vi "Initial Connection.vi"(0 "Systems Config Path":path=path "C:/Users/gtetil/Documents/Projects/TI-cDAQ/Source/Systems Config.ini", 5 "Error IN":errorcluster) -> (14 "Close Program":bool, 15 "Connected":bool, 16 "System Ref":tag, 17 "Selected System":T1, 19 "Error OUT":errorcluster)   [LabVIEW 2023]
uses:
  Type Defs and Controls/System Buttons.ctl
  Type Defs and Controls/System Button.ctl
  Type Defs and Controls/System Config.ctl
  Type Defs and Controls/Systems Config.ctl
  <vilib>/Utility/cursorutil.llb/Set Cursor (Icon Pict).vi
  <vilib>/Utility/config.llb/NI_LVConfig.lvlib
  <userlib>/_OpenG.lib/variantconfig/variantconfig.llb/openg_variant_configuration_file.lvlib
panel:
  out "Abort 2":bool
  in  "Exit":bool
  in  "Abort":bool
  out "Connecting Indicator":string="Connecting..."
  in  "Tab Control":enum32{"Main", "Connecting"}(tab)
  in  "Systems":T2={"System 1"={"System Button"=FALSE, "Description"="Deformation"}, "System 2"={"System Button"=FALSE, "Description"="Standard"}, "System 3"={"System Button"=FALSE, "Description"="Standard"}, "System 4"={"System Button"=FALSE, "Description"="Standard"}, "System 5"={"System Button"=FALSE, "Description"="Standard XT"}, "System 6"={"System Button"=FALSE, "Description"=""}, "System 7"={"System Button"=FALSE, "Description"=""}, "System 8"={"System Button"=FALSE, "Description"=""}, "System 9"={"System Button"=FALSE, "Description"=""}}
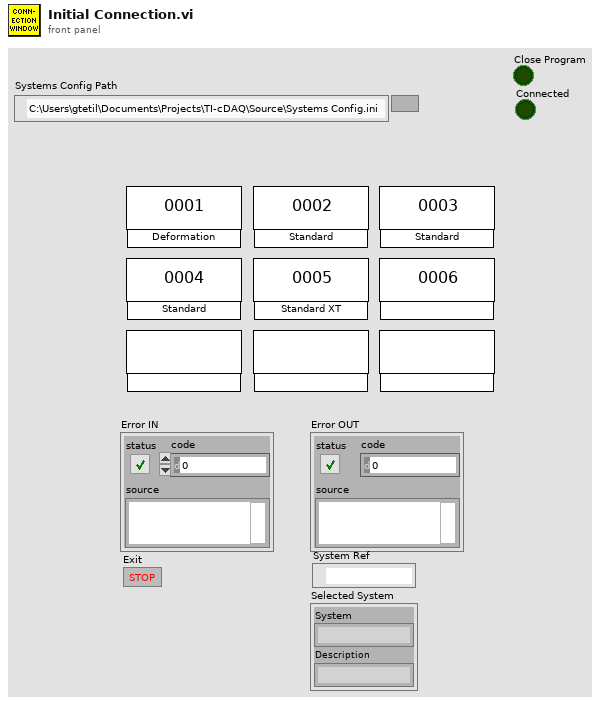
[diagram p1: front panel]
types:
  T1 = typedef "System Config.ctl" = cluster{"System":string, "Description":string}
  T2 = typedef "System Buttons.ctl" = cluster{"System 1":T3, "System 2":T3, "System 3":T3, "System 4":T3, "System 5":T3, "System 6":T3, "System 7":T3, "System 8":T3, "System 9":T3}
  T3 = typedef "System Button.ctl" = cluster{"System Button":bool, "Description":string}
  T4 = typedef "Systems Config.ctl" = cluster{"System 1":T1, "System 2":T1, "System 3":T1, "System 4":T1, "System 5":T1, "System 6":T1, "System 7":T1, "System 8":T1, "System 9":T1}
  T5 = cluster{"Error IN":errorcluster, "Systems Config Path":path, "Systems Config":T4, "Selected System":T1, "Close Program":bool, "Connected":bool, "System Ref":tag}
  T6 = enum8{"Enabled", "Disabled", "Disabled and Grayed Out"}
  T7 = typedef "NI_LVConfig.lvlib/Config Data RefNum.ctl" = refnum<k1>
  T8 = enum32{"invalid app kind", "Development System", "Run Time System", "Student Edition", "Embedded LabVIEW", "Evaluation", "Custom"}
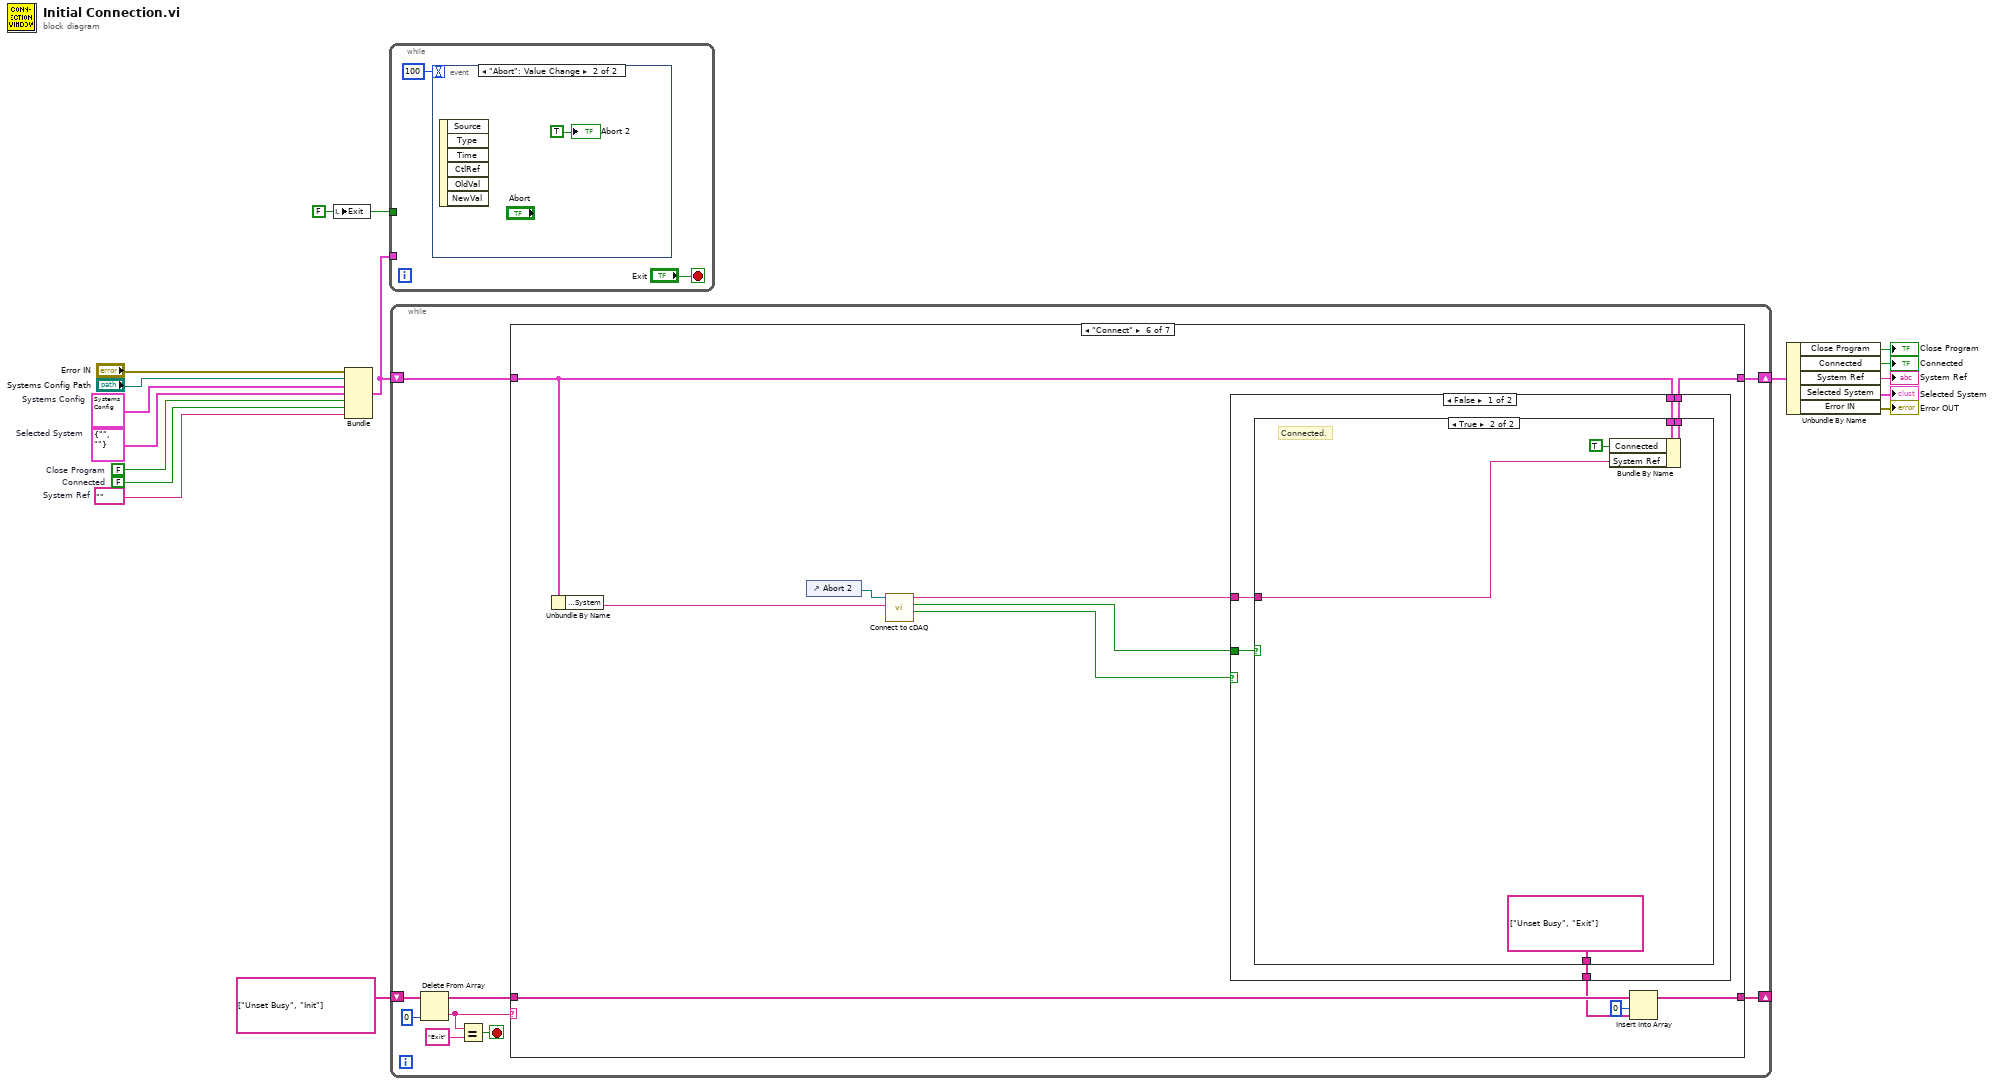
[diagram p0: block diagram]
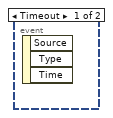
[diagram p2: hidden frame]
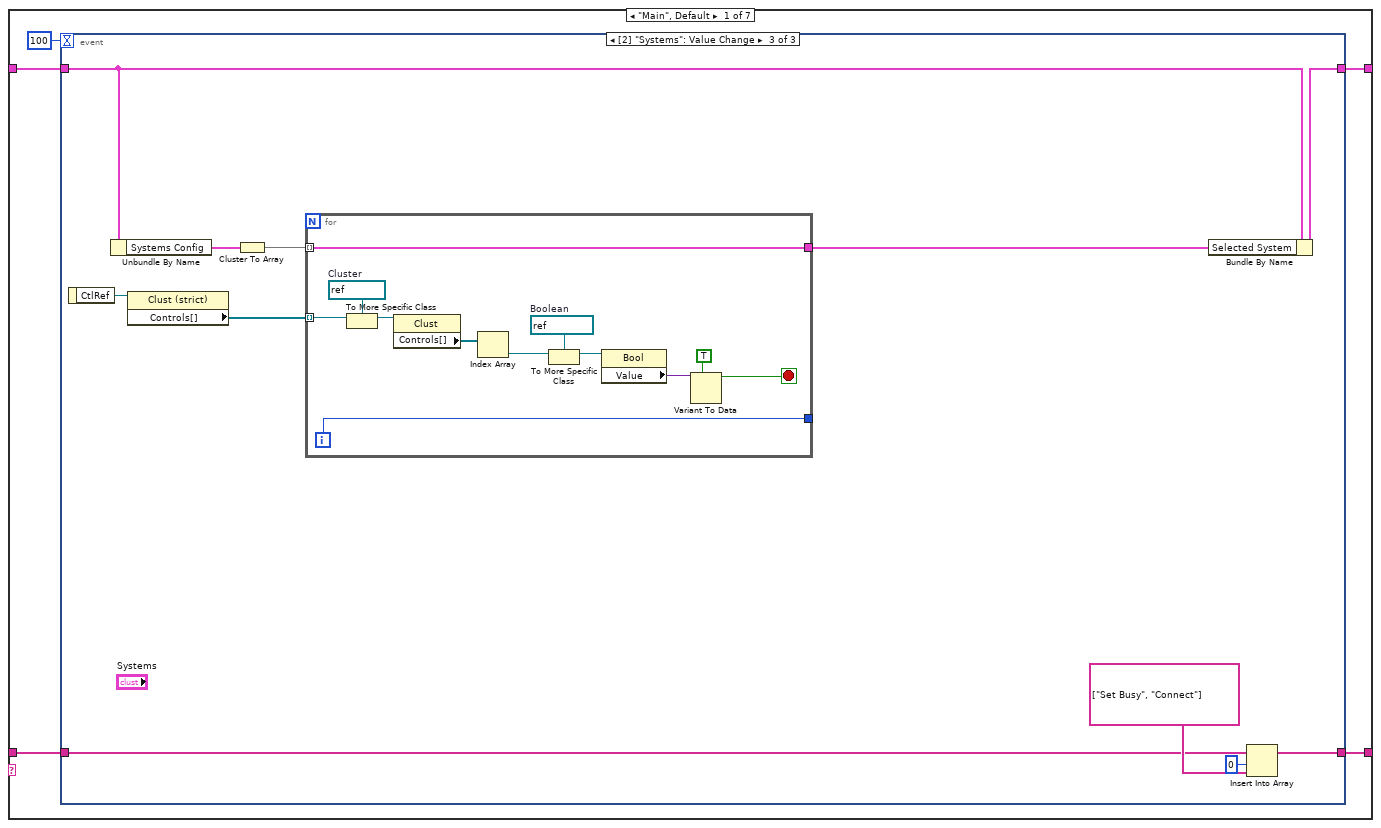
[diagram p3: hidden frame]
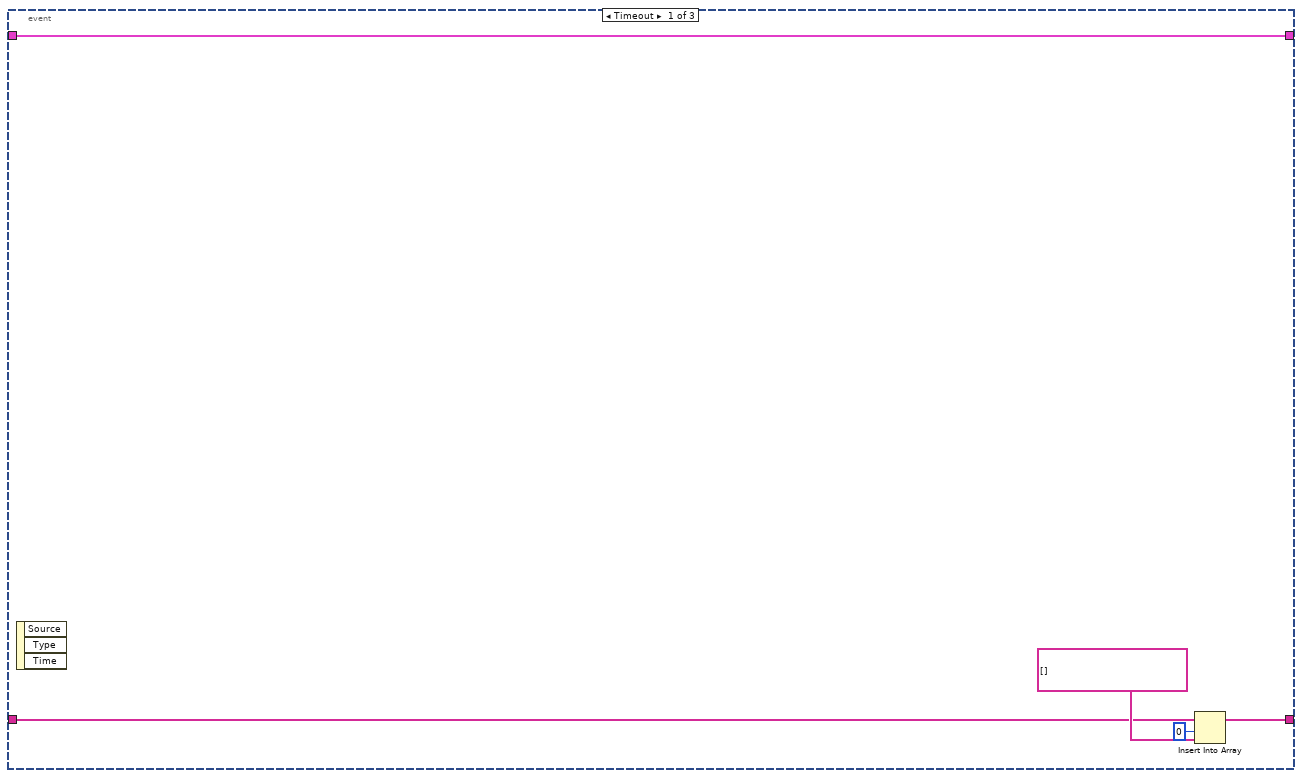
[diagram p4: hidden frame]
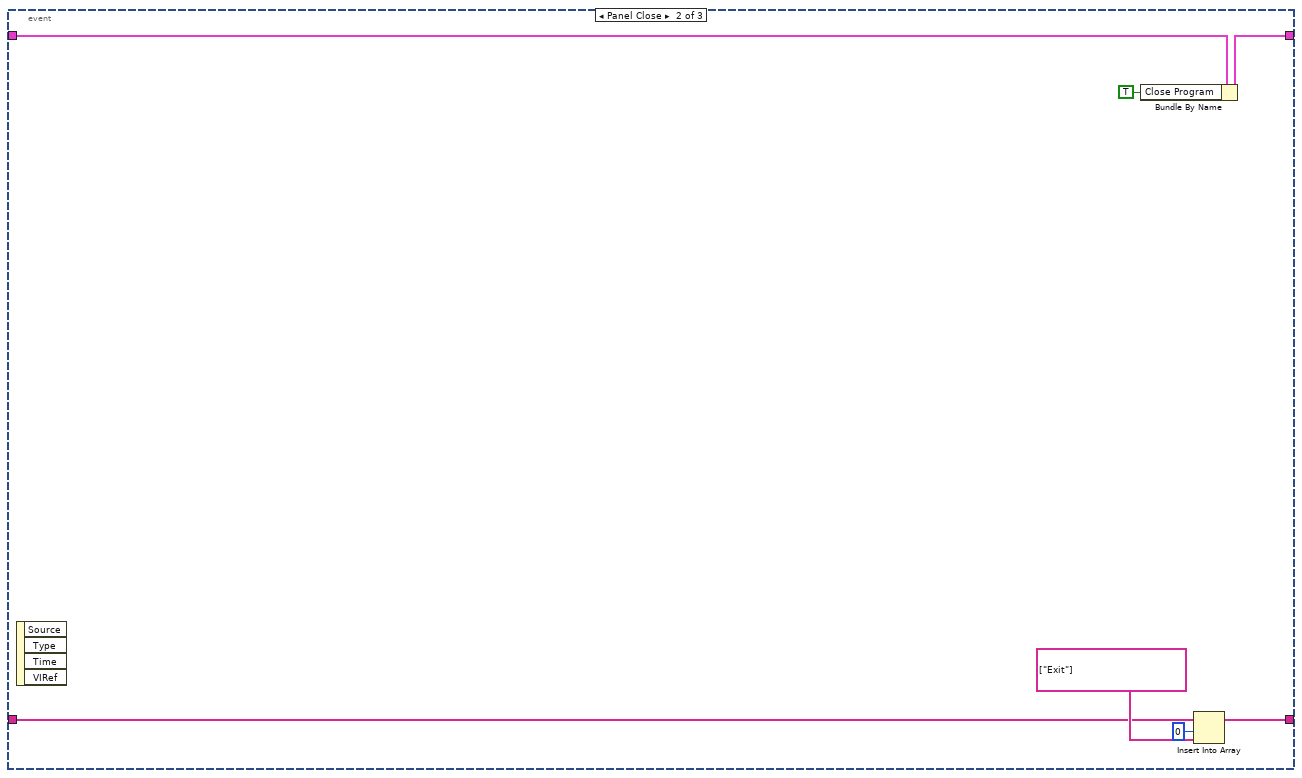
[diagram p5: hidden frame]
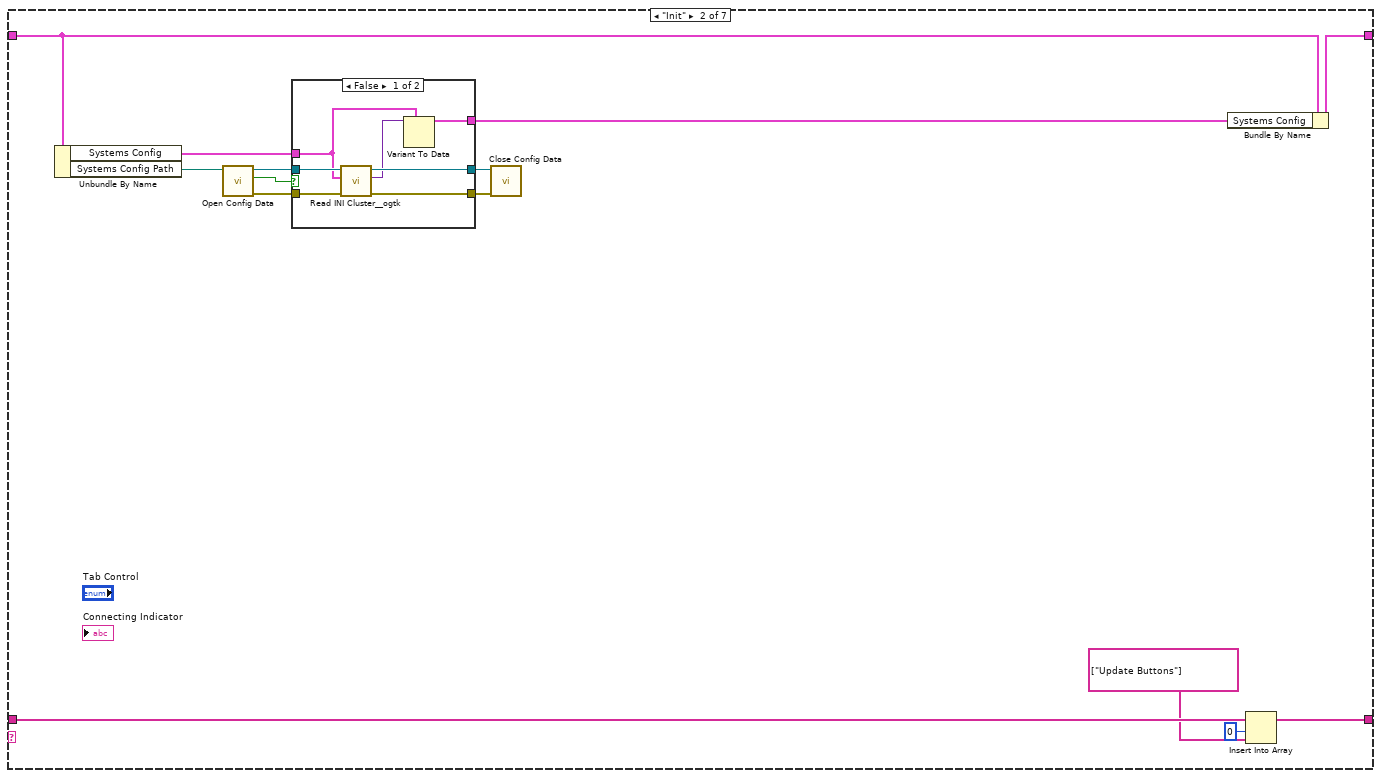
[diagram p6: hidden frame]
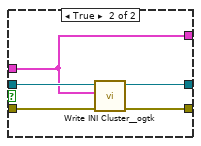
[diagram p7: hidden frame]
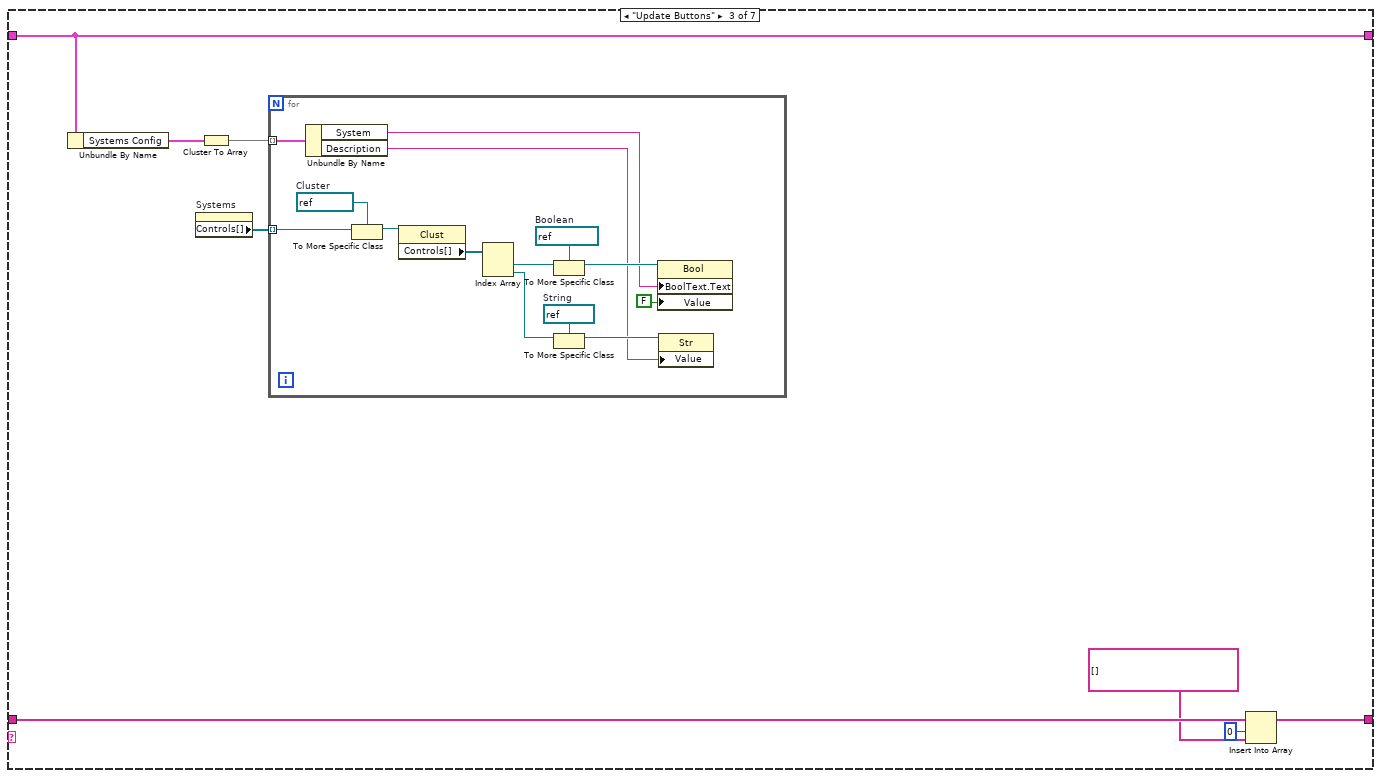
[diagram p8: hidden frame]
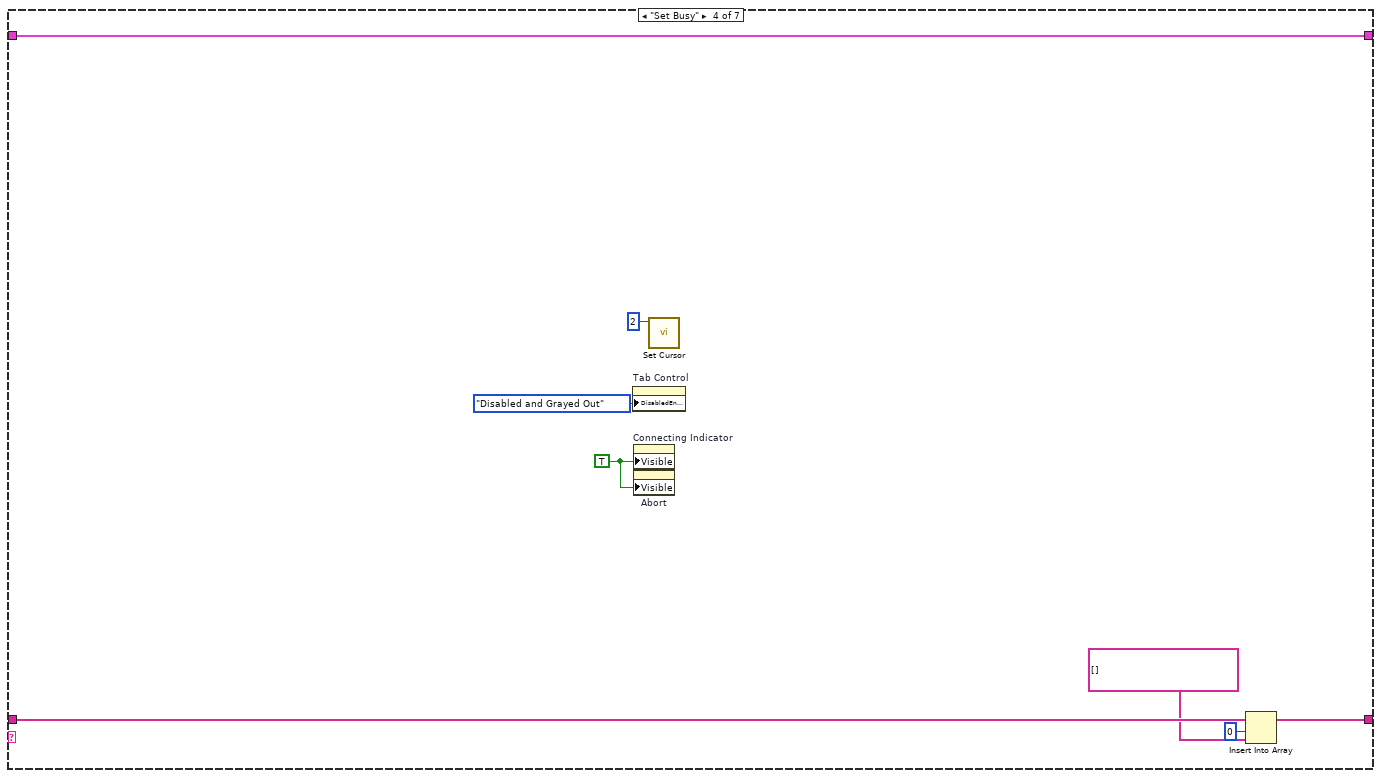
[diagram p9: hidden frame]
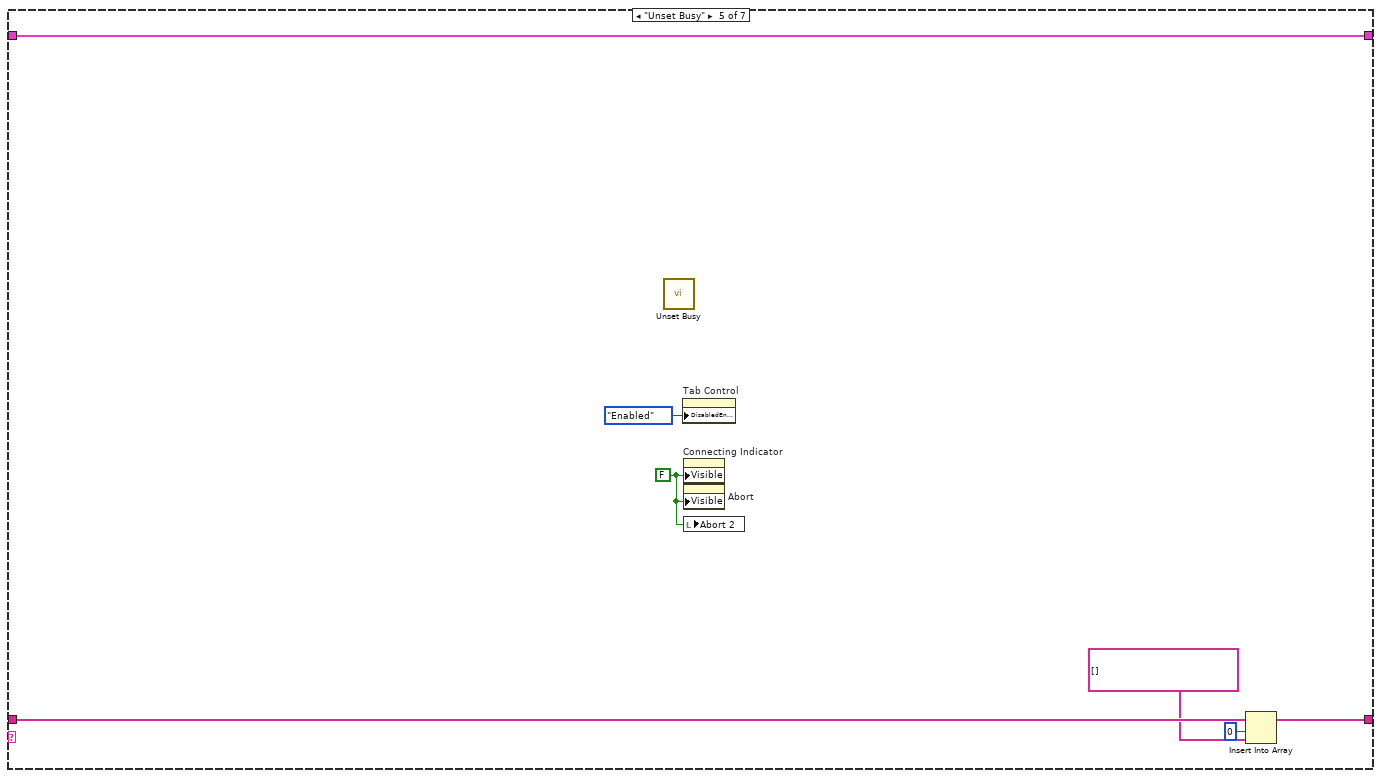
[diagram p10: hidden frame]
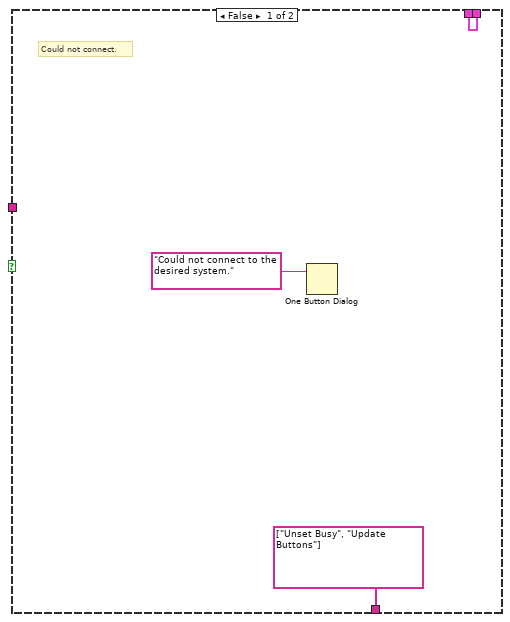
[diagram p11: hidden frame]
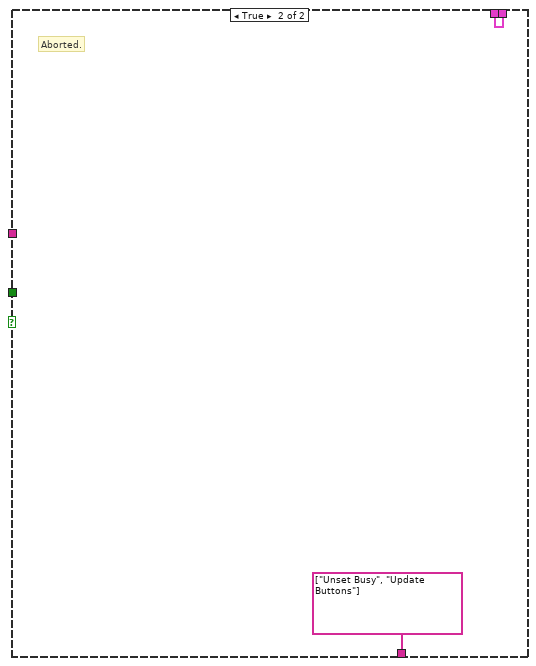
[diagram p12: hidden frame]
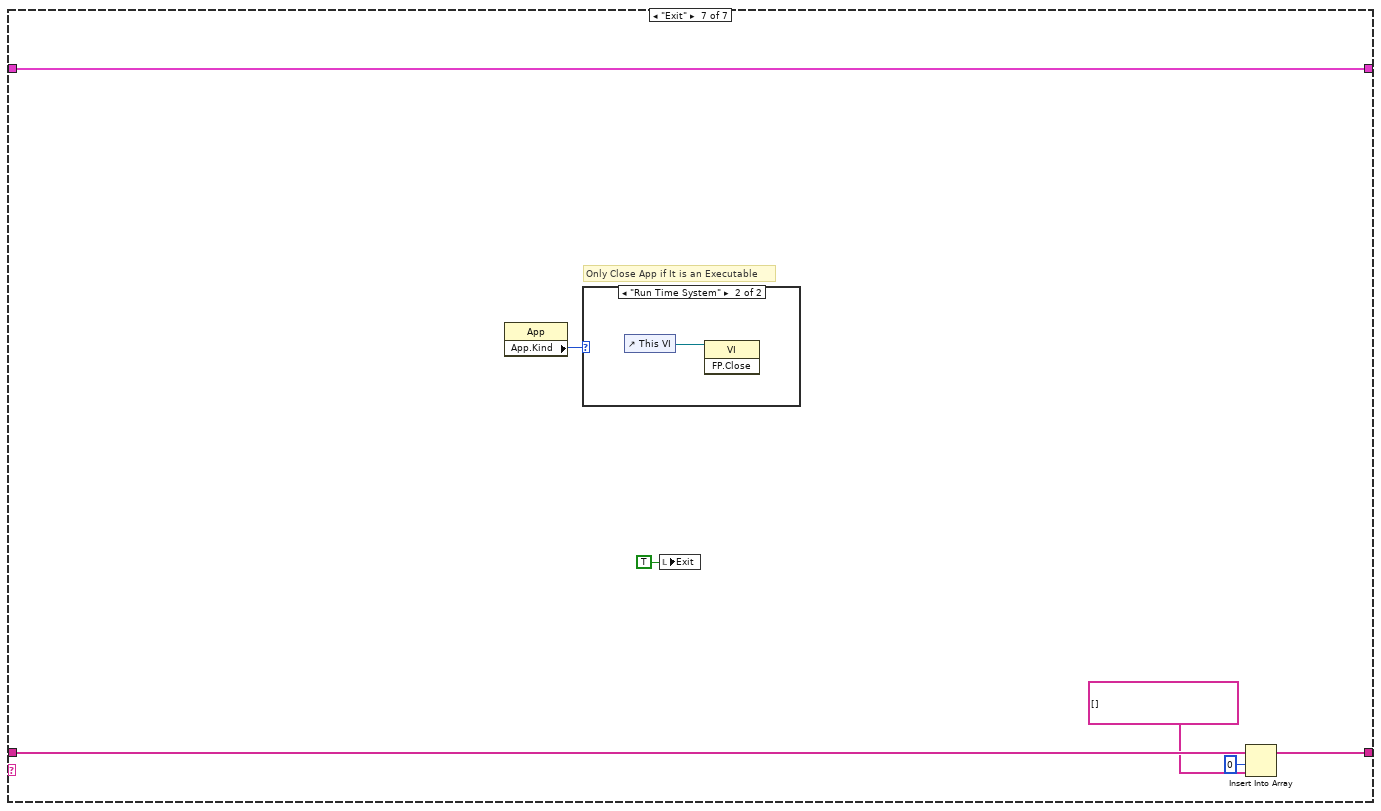
[diagram p13: hidden frame]
diagram:
  w1 = FALSE ("Exit")
  w5 = tag ""  # System Ref
  w8 = FALSE  # Connected
  w11 = FALSE  # Close Program
  w12 = T1 {"System"="", "Description"=""}  # Selected System
  w13 = T4 {"System 1"={"System"="", "Description"=""}, "System 2"={"System"="", "Description"=""}, "System 3"={"System"="", "Description"=""}, "System 4"={"System"="", "Description"=""}, "System 5"={"System"="", "Description"=""}, "System 6"={"System"="", "Description"=""}, "System 7"={"System"="", "Description"=""}, "System 8"={"System"="", "Description"=""}, "System 9"={"System"="", "Description"=""}}  # Systems Config
  n1 = local write "Exit"(w1) -> ()
  n2 = Bundle("Error IN"="Error IN", "Systems Config Path"="Systems Config Path", "Systems Config"=w13, "Selected System"=w12, "Close Program"=w11, "Connected"=w8, "System Ref"=w5) -> (w2:T5)  [unwired: 1 in]
  n3 = while {
    tunnel: w2 -> [_]
    tunnel: w1 -> [_]
    stop <- "Exit" stop-if-true
    n4 = event shown="[1] \"Abort\": Value Change" {
      selector: _ -> [_ _]
      dyn-events: _ -> [_ _]
      timeout: 100 -> [_ _]
      event Timeout {
        n5 = event-data() -> ()  [unwired: 1 in, 3 out]
      }
      event "Abort": Value Change {
        n6 = event-data() -> ()  [unwired: 1 in, 6 out]
        "Abort 2" <- TRUE ("Abort 2")
      }
    }
  }
  n7 = while {
    shift-right: [w23] -> _
    shift-left: string[] ["Unset Busy", "Init"] -> [w28]
    shift-right: [w20] -> w10
    shift-left: w2 -> [w21]
    stop <- w24 stop-if-true
    n8 = Delete From Array(array=w28, index=0 ("length")) -> (deleted portion=w25:string, array with subset deleted=w22:string[])  [unwired: 1 in]
    n9 = Equal?(x=w25, y="Exit") -> (x = y?=w24:bool)
    n10 = case shown="\"Connect\"" w25 {
      tunnel: [w29 w81 w102 w124 w131 w142 w164] -> w23
      tunnel: w22 -> [w30 w80 w101 w123 w130 w141 w163]
      tunnel: w21 -> [w33 w77 w98 w120 w127 w136 w160]
      tunnel: [w32 w82 w98 w120 w127 w137 w160] -> w20
      frame "Main", Default {
        n11 = event shown="[2] \"Systems\": Value Change" {
          selector: _ -> [_ _ _]
          dyn-events: _ -> [_ _ _]
          timeout: 100 -> [_ _ _]
          tunnel: w33 -> [w38 w40 w49]
          tunnel: [w38 w41 w50] -> w32
          tunnel: w30 -> [w35 w42 w54]
          tunnel: [w34 w43 w53] -> w29
          event Timeout {
            n12 = event-data() -> ()  [unwired: 1 in, 3 out]
            n13 = Insert Into Array(array=w35, index=0, new element=string[] []) -> (w34:string[])
          }
          event Panel Close {
            n14 = event-data() -> ()  [unwired: 1 in, 4 out]
            n15 = Bundle By Name(cluster=w40, "Close Program"=TRUE) -> (w41:T5)
            n16 = Insert Into Array(array=w42, index=0, new element=string[] ["Exit"]) -> (w43:string[])
          }
          event Value Change {
            n17 = event-data() -> ("CtlRef"=w52:refnum<vi>)  [unwired: 1 in]
            n18 = Unbundle By Name(w49) -> ("Systems Config"=w48:T4)
            n19 = property class="Clust (strict)"(reference=w52) -> ("Controls[]"=w51:refnum<vi>[])  [unwired: 1 in, 2 out]
            n20 = Cluster To Array(cluster=w48) -> (array=w47:T1[])
            n21 = for {
              tunnel: w51 -> [w62] mode=indexing
              tunnel: [w58] -> _
              tunnel: w47 -> [w57] mode=indexing
              tunnel: [w57] -> w46
              i -> [w58]
              stop <- w59 stop-if-true
              w64 = refnum<vi> refnum  # Boolean
              w63 = refnum<vi> refnum  # Cluster
              n22 = To More Specific Class(target class=w63, reference=w62) -> (specific class reference=w68:refnum<vi>)  [unwired: 1 in, 1 out]
              n23 = property class="Clust"(reference=w68) -> ("Controls[]"=w67:refnum<vi>[])  [unwired: 1 in, 2 out]
              n24 = Index Array(array=w67) -> (element=w66:refnum<vi>)  [unwired: 1 in]
              n25 = To More Specific Class(target class=w64, reference=w66) -> (specific class reference=w65:refnum<vi>)  [unwired: 1 in, 1 out]
              n26 = property class="Bool"(reference=w65) -> ("Value"=w61:variant)  [unwired: 1 in, 2 out]
              n27 = Variant To Data(type=TRUE, Variant=w61) -> (data=w59:bool)  [unwired: 1 in, 1 out]
            }
            n28 = Bundle By Name(cluster=w49, "Selected System"=w46) -> (w50:T5)
            n29 = Insert Into Array(array=w54, index=0, new element=string[] ["Set Busy", "Connect"]) -> (w53:string[])
          }
        }
      }
      frame "Init" {
        n30 = Unbundle By Name(w77) -> ("Systems Config"=w71:T4, "Systems Config Path"=w76:path)
        n31 = call <vilib>:"Open Config Data.vi"("configuration file path"=w76) -> ("error out"=w75:errorcluster, "file created?"=w69:bool, "refnum"=w74:T7)  [unwired: 8 in]
        n32 = case shown="False" w69 {
          tunnel: w75 -> [w89 w93]
          tunnel: w74 -> [w88 w94]
          tunnel: [w87 w92] -> w73
          tunnel: [w86 w91] -> w72
          tunnel: w71 -> [w85 w90]
          tunnel: [w83 w90] -> w70
          frame False {
            n33 = call <userlib>:"Read INI Cluster__ogtk.vi"("error in (no error)"=w89, "INI Fomatted Cluster Type"=w85, "refnum"=w88) -> ("error out"=w86:errorcluster, "INI Fomatted Cluster"=w84:variant, "dup refnum"=w87:T7)  [unwired: 4 in, 2 out]
            n34 = Variant To Data(type=w85, Variant=w84) -> (data=w83:T4)  [unwired: 1 in, 1 out]
          }
          frame True {
            n35 = call <userlib>:"Write INI Cluster__ogtk.vi"("error in (no error)"=w93, "INI Fomatted Cluster"=w90, "refnum"=w94) -> ("error out"=w91:errorcluster, "dup refnum"=w92:T7)  [unwired: 7 in]
          }
        }
        n36 = call <vilib>:"Close Config Data.vi"("error in (no error)"=w72, "refnum"=w73) -> ()  [unwired: 8 in, 2 out]
        n37 = Bundle By Name(cluster=w77, "Systems Config"=w70) -> (w82:T5)
        n38 = Insert Into Array(array=w80, index=0, new element=string[] ["Update Buttons"]) -> (w81:string[])
      }
      frame "Update Buttons" {
        n39 = Unbundle By Name(w98) -> ("Systems Config"=w97:T4)
        n40 = property on="Systems" class="Clust (strict)"() -> ("Controls[]"=w95:refnum<vi>[])  [unwired: 2 in, 2 out]
        n41 = Cluster To Array(cluster=w97) -> (array=w96:T1[])
        n42 = for {
          tunnel: w96 -> [w116] mode=indexing
          tunnel: w95 -> [w113] mode=indexing
          w109 = refnum<vi> refnum  # String
          w110 = refnum<vi> refnum  # Boolean
          w112 = refnum<vi> refnum  # Cluster
          n43 = Unbundle By Name(w116) -> ("System"=w105:string, "Description"=w104:string)
          n44 = To More Specific Class(target class=w112, reference=w113) -> (specific class reference=w115:refnum<vi>)  [unwired: 1 in, 1 out]
          n45 = property class="Clust"(reference=w115) -> ("Controls[]"=w114:refnum<vi>[])  [unwired: 1 in, 2 out]
          n46 = Index Array(array=w114) -> (element #1=w111:refnum<vi>, element #2=w108:refnum<vi>)  [unwired: 2 in]
          n47 = To More Specific Class(target class=w110, reference=w111) -> (specific class reference=w107:refnum<vi>)  [unwired: 1 in, 1 out]
          n48 = To More Specific Class(target class=w109, reference=w108) -> (specific class reference=w106:refnum<vi>)  [unwired: 1 in, 1 out]
          n49 = property class="Bool"(reference=w107, "BoolText.Text"=w105, "Value"=FALSE) -> ()  [unwired: 1 in, 2 out]
          n50 = property class="Str"(reference=w106, "Value"=w104) -> ()  [unwired: 1 in, 2 out]
        }
        n51 = Insert Into Array(array=w101, index=0, new element=string[] []) -> (w102:string[])
      }
      frame "Set Busy" {
        w118 = TRUE ("Visible")
        n52 = property on="Tab Control" class="TabCtl (strict)"("DisabledEnum"=T6."Disabled and Grayed Out" ("Disabled")) -> ()  [unwired: 2 in, 2 out]
        n53 = property on="Connecting Indicator" class="Str"("Visible"=w118) -> ()  [unwired: 2 in, 2 out]
        n54 = property on="Abort" class="Bool"("Visible"=w118) -> ()  [unwired: 2 in, 2 out]
        n55 = call-poly <vilib>:"Set Cursor.vi"("icon"=u16 2) -> ()  [unwired: 9 in, 2 out]
        n56 = Insert Into Array(array=w123, index=0, new element=string[] []) -> (w124:string[])
      }
      frame "Unset Busy" {
        w125 = FALSE ("Visible")
        n57 = call <vilib>:"Unset Busy.vi"() -> ()  [unwired: 11 in, 1 out]
        n58 = property on="Tab Control" class="TabCtl (strict)"("DisabledEnum"=T6."Enabled" ("Disabled")) -> ()  [unwired: 2 in, 2 out]
        n59 = property on="Connecting Indicator" class="Str"("Visible"=w125) -> ()  [unwired: 2 in, 2 out]
        n60 = property on="Abort" class="Bool"("Visible"=w125) -> ()  [unwired: 2 in, 2 out]
        n61 = local write "Abort 2"(w125) -> ()
        n62 = Insert Into Array(array=w130, index=0, new element=string[] []) -> (w131:string[])
      }
      frame "Connect" {
        n63 = Unbundle By Name(w136) -> ("Selected System.System"=w133:string)
        n64 = control-ref of="Abort 2"() -> (w132:refnum<vi>)
        n65 = call "Connect to cDAQ.vi"("System"=w133, "Abort Ref"=w132) -> ("Abort"=w134:bool, "Connected?"=w138:bool, "System Ref"=w135:tag)  [unwired: 7 in]
        n66 = case shown="False" w134 {
          tunnel: [w147 string[] ["Unset Busy", "Update Buttons"]] -> w140
          tunnel: w138 -> [w146 _]
          tunnel: [w145 w157] -> w137
          tunnel: w136 -> [w144 w157]
          tunnel: w135 -> [w143 _]
          frame False {
            n67 = case shown="True" w146 {
              tunnel: [string[] ["Unset Busy", "Update Buttons"] string[] ["Unset Busy", "Exit"]] -> w147
              tunnel: w144 -> [w150 w154]
              tunnel: [w150 w153] -> w145
              tunnel: w143 -> [_ w151]
              frame False {
                # "Could not connect."
                n68 = One Button Dialog(message="Could not connect to the desired system.") -> ()  [unwired: 1 in, 1 out]
              }
              frame True {
                # "Connected."
                n69 = Bundle By Name(cluster=w154, "Connected"=TRUE, "System Ref"=w151) -> (w153:T5)
              }
            }
          }
          frame True {
            # "Aborted."
          }
        }
        n70 = Insert Into Array(array=w141, index=0, new element=w140) -> (w142:string[])
      }
      frame "Exit" {
        # "Only Close App if It is an Executable"
        n71 = property class="App"() -> ("App.Kind"=w158:T8)  [unwired: 2 in, 2 out]
        n72 = case shown="\"Run Time System\"" w158 {
          frame Default {
          }
          frame "Run Time System" {
            n73 = control-ref of="This VI"() -> (w165:refnum<vi>)
            n74 = invoke class="VI" method="FP.Close"(reference=w165) -> ()  [unwired: 2 in, 3 out]
          }
        }
        n75 = local write "Exit"(TRUE ("Exit")) -> ()
        n76 = Insert Into Array(array=w163, index=0, new element=string[] []) -> (w164:string[])
      }
    }
  }
  n77 = Unbundle By Name(w10) -> ("Close Program"=→"Close Program":bool, "Connected"=→"Connected":bool, "System Ref"=→"System Ref":tag, "Selected System"=→"Selected System":T1, "Error IN"=→"Error OUT":errorcluster)
